vi "Insert.vi"(6 "commandTimeout":i32, 7 "SqlMapper in":refnum<class "SqlMapper.lvclass">, 8 "error in (no error)":errorcluster, 9 "DynamicParameters":refnum<class "DynamicParameters.lvclass">, 10 "tableName":string, 11 "PostgresqlConnection in":refnum<class "PostgresqlConnection.lvclass">) -> (0 "error out":errorcluster, 2 "id":variant, 3 "PostgresqlConnection out":refnum<class "PostgresqlConnection.lvclass">, 5 "SqlMapper out":refnum<class "SqlMapper.lvclass">)   [LabVIEW 2018]
uses:
  PostgresqlConnection.lvclass
  Dapper/SqlMapper/SqlMapper.lvclass
  Dapper/DynamicParameters/DynamicParameters.lvclass
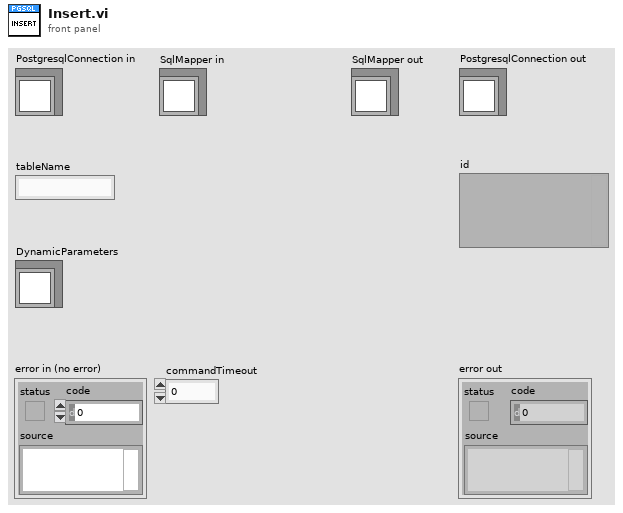
[diagram p1: front panel]
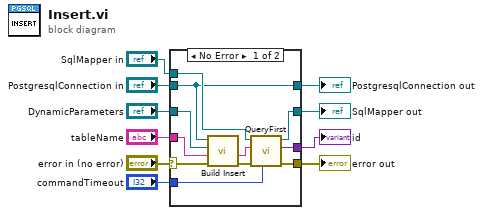
[diagram p0: block diagram]
diagram:
  n1 = case shown="No Error" "error in (no error)" {
    selector: "error in (no error)" -> [w14 w24]
    tunnel: [w17 w24] -> w1
    tunnel: [w12 w23] -> w10
    tunnel: "PostgresqlConnection in" -> [w12 w23]
    tunnel: "SqlMapper in" -> [w19 w22]
    tunnel: "DynamicParameters" -> [w21 _]
    tunnel: "commandTimeout" -> [w11 _]
    tunnel: [w18 w22] -> w9
    tunnel: "tableName" -> [w20 _]
    tunnel: [w16 _] -> w2
    frame No Error {
      n2 = call-dynamic "Build Insert.vi"("error in (no error)"=w14, "tableName"=w20, "DynamicParameters in"=w21, "PostgresqlConnection in"=w12) -> ("error out"=w13:errorcluster, "QueryString Out"=w15:string)  [unwired: 5 in, 1 out]
      n3 = call-dynamic "QueryFirst.vi"("commandTimeout in"=w11, "error in (no error)"=w13, "sql"=w15, "SqlMapper in"=w19) -> ("error out"=w17:errorcluster, "Value"=w16:variant, "SqlMapper out"=w18:refnum<class "SqlMapper.lvclass">)  [unwired: 5 in]
    }
    frame Error {
    }
  }
  "error out" <- w1
  "PostgresqlConnection out" <- w10
  "id" <- w2
  "SqlMapper out" <- w9
